vi "Plotmatrix Marker Property.vi"(6 "Update?":bool, 8 "error in (no error)":errorcluster, 9 "Scale Array In":T1, 11 "Single XY Plot In":refnum<vi>) -> (0 "error out":errorcluster, 3 "Single XY Plot Out":refnum<vi>)   [LabVIEW 2017, in "XY Plot Matrix.lvclass"]
uses:
  <vilib>/Math Plots/2D Math Plots/XY Plot Matrix/XY Plot Matrix/XY Plot Matrix.lvclass
  <vilib>/Math Plots/2D Math Plots/2D Plot/2D Plot/Typedef/Scale Array.ctl
  <vilib>/Math Plots/2D Math Plots/2D Plot/2D Plot/Typedef/Scale Cluster.ctl
  <vilib>/Utility/miscctls.llb/LVOffsetAndMultiplierTypeDef.ctl
  <vilib>/Math Plots/2D Math Plots/2D Plot/2D Plot/2D Plot.lvclass
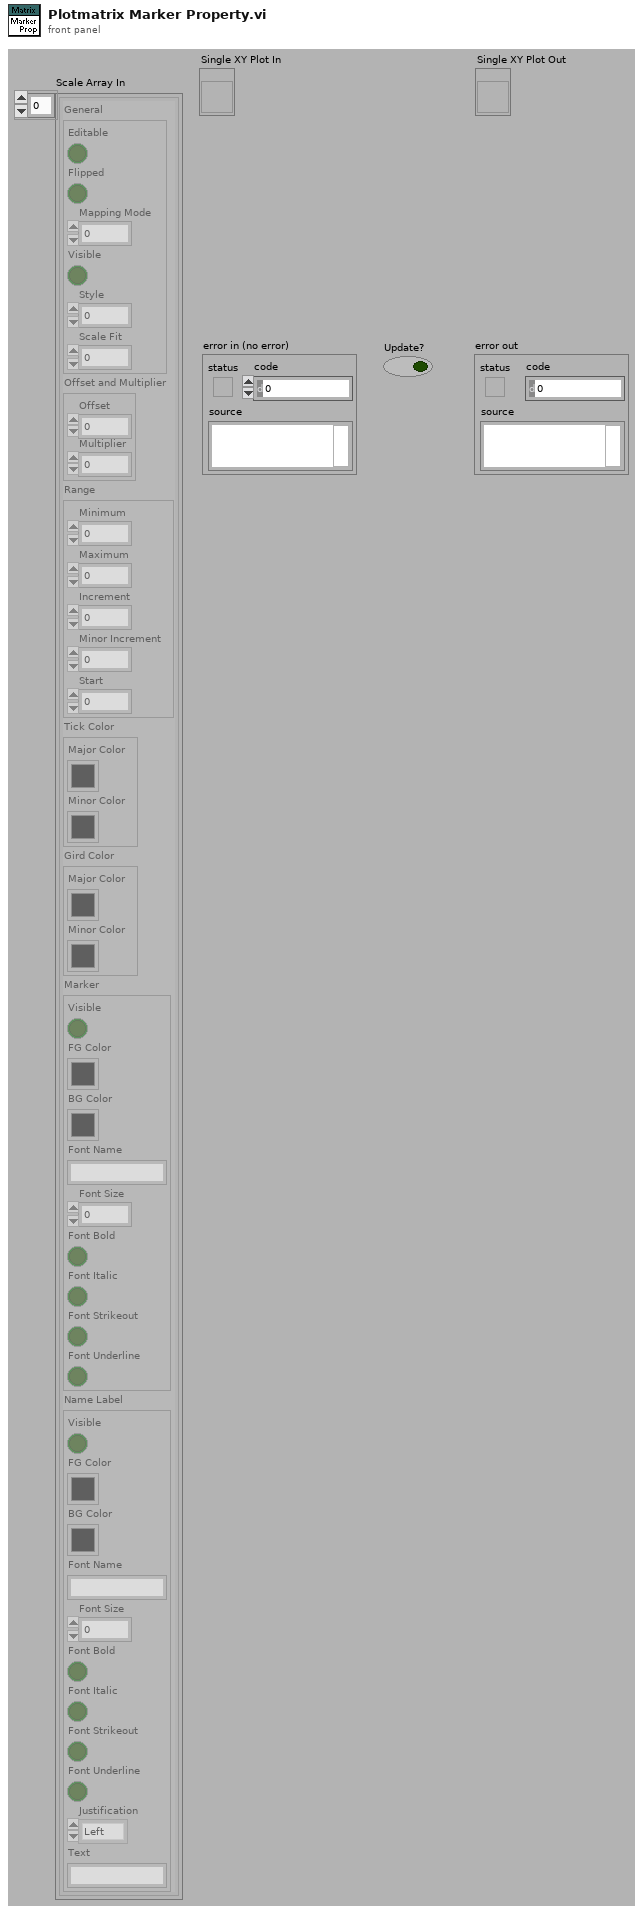
[diagram p1: front panel]
types:
  T1 = typedef "2D Plot.lvclass/Scale Array.ctl" = T2[]
  T2 = typedef "2D Plot.lvclass/Scale Cluster.ctl" = cluster{"General":cluster{"Editable":bool, "Flipped":bool, "Mapping Mode":u8, "Visible":bool, "Style":u8, "Scale Fit":u8}, "Offset and Multiplier":T3, "Range":cluster{"Minimum":dbl, "Maximum":dbl, "Increment":dbl, "Minor Increment":dbl, "Start":dbl}, "Tick Color":cluster{"Major Color":u32, "Minor Color":u32}, "Gird Color":cluster{"Major Color":u32, "Minor Color":u32}, "Marker":cluster{"Visible":bool, "FG Color":u32, "BG Color":u32, "Font Name":string, "Font Size":u32, "Font Bold":bool, "Font Italic":bool, "Font Strikeout":bool, "Font Underline":bool}, "Name Label":cluster{"Visible":bool, "FG Color":u32, "BG Color":u32, "Font Name":string, "Font Size":u32, "Font Bold":bool, "Font Italic":bool, "Font Strikeout":bool, "Font Underline":bool, "Justification":enum16{"Left", "Center", "Right"}, "Text":string}}
  T3 = typedef "LVOffsetAndMultiplierTypeDef.ctl" = cluster{"Offset":dbl, "Multiplier":dbl}
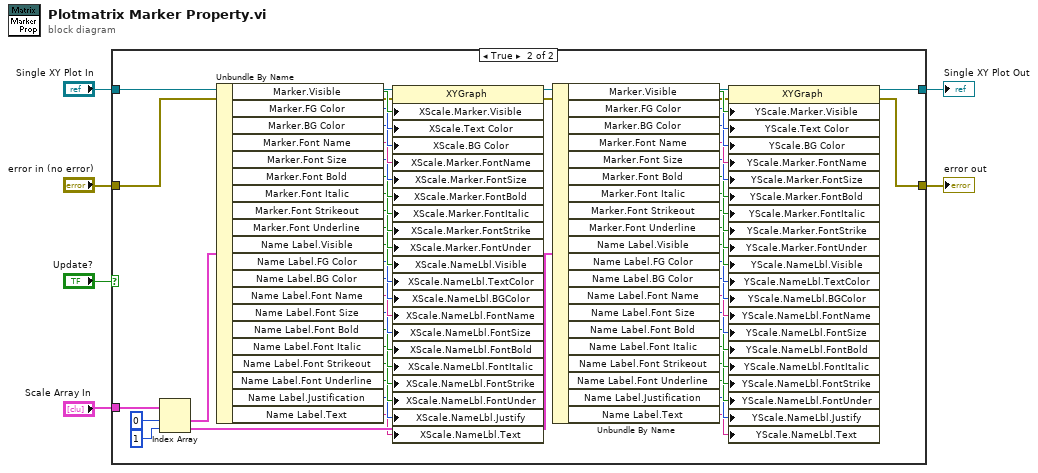
[diagram p0: block diagram]
diagram:
  n1 = case shown="True" "Update?" {
    tunnel: "Scale Array In" -> [_ w59]
    tunnel: "Single XY Plot In" -> [w8 w36]
    tunnel: "error in (no error)" -> [w7 w35]
    tunnel: [w8 w12] -> w3
    tunnel: [w7 w11] -> w2
    frame False {
    }
    frame True {
      n2 = Index Array(array=w59, index #1=0 ("index"), index #2=1 ("index")) -> (element #1=w58:T2, element #2=w57:T2)
      n3 = Unbundle By Name(w58) -> ("Marker.Visible"=w56:bool, "Marker.FG Color"=w55:u32, "Marker.BG Color"=w54:u32, "Marker.Font Name"=w53:string, "Marker.Font Size"=w52:u32, "Marker.Font Bold"=w51:bool, "Marker.Font Italic"=w50:bool, "Marker.Font Strikeout"=w49:bool, "Marker.Font Underline"=w48:bool, "Name Label.Visible"=w47:bool, "Name Label.FG Color"=w46:u32, "Name Label.BG Color"=w45:u32, "Name Label.Font Name"=w44:string, "Name Label.Font Size"=w43:u32, "Name Label.Font Bold"=w42:bool, "Name Label.Font Italic"=w41:bool, "Name Label.Font Strikeout"=w40:bool, "Name Label.Font Underline"=w39:bool, "Name Label.Justification"=w38:enum16{"Left", "Center", "Right"}, "Name Label.Text"=w37:string)
      n4 = property class="XYGraph"(reference=w36, error in=w35, "XScale.Marker.Visible"=w56, "XScale.Text Color"=w55, "XScale.BG Color"=w54, "XScale.Marker.FontName"=w53, "XScale.Marker.FontSize"=w52, "XScale.Marker.FontBold"=w51, "XScale.Marker.FontItalic"=w50, "XScale.Marker.FontStrike"=w49, "XScale.Marker.FontUnder"=w48, "XScale.NameLbl.Visible"=w47, "XScale.NameLbl.TextColor"=w46, "XScale.NameLbl.BGColor"=w45, "XScale.NameLbl.FontName"=w44, "XScale.NameLbl.FontSize"=w43, "XScale.NameLbl.FontBold"=w42, "XScale.NameLbl.FontItalic"=w41, "XScale.NameLbl.FontStrike"=w40, "XScale.NameLbl.FontUnder"=w39, "XScale.NameLbl.Justify"=w38, "XScale.NameLbl.Text"=w37) -> (reference out=w14:refnum<vi>, error out=w13:errorcluster)
      n5 = Unbundle By Name(w57) -> ("Marker.Visible"=w34:bool, "Marker.FG Color"=w33:u32, "Marker.BG Color"=w32:u32, "Marker.Font Name"=w31:string, "Marker.Font Size"=w30:u32, "Marker.Font Bold"=w29:bool, "Marker.Font Italic"=w28:bool, "Marker.Font Strikeout"=w27:bool, "Marker.Font Underline"=w26:bool, "Name Label.Visible"=w25:bool, "Name Label.FG Color"=w24:u32, "Name Label.BG Color"=w23:u32, "Name Label.Font Name"=w22:string, "Name Label.Font Size"=w21:u32, "Name Label.Font Bold"=w20:bool, "Name Label.Font Italic"=w19:bool, "Name Label.Font Strikeout"=w18:bool, "Name Label.Font Underline"=w17:bool, "Name Label.Justification"=w16:enum16{"Left", "Center", "Right"}, "Name Label.Text"=w15:string)
      n6 = property class="XYGraph"(reference=w14, error in=w13, "YScale.Marker.Visible"=w34, "YScale.Text Color"=w33, "YScale.BG Color"=w32, "YScale.Marker.FontName"=w31, "YScale.Marker.FontSize"=w30, "YScale.Marker.FontBold"=w29, "YScale.Marker.FontItalic"=w28, "YScale.Marker.FontStrike"=w27, "YScale.Marker.FontUnder"=w26, "YScale.NameLbl.Visible"=w25, "YScale.NameLbl.TextColor"=w24, "YScale.NameLbl.BGColor"=w23, "YScale.NameLbl.FontName"=w22, "YScale.NameLbl.FontSize"=w21, "YScale.NameLbl.FontBold"=w20, "YScale.NameLbl.FontItalic"=w19, "YScale.NameLbl.FontStrike"=w18, "YScale.NameLbl.FontUnder"=w17, "YScale.NameLbl.Justify"=w16, "YScale.NameLbl.Text"=w15) -> (reference out=w12:refnum<vi>, error out=w11:errorcluster)
    }
  }
  "Single XY Plot Out" <- w3
  "error out" <- w2
